vi "Set Command Factory.vi"(10 "commandFactory":refnum<class "Command Factory.lvclass">, 11 "Model in":refnum<class "Model.lvclass">) -> (3 "Model out":refnum<class "Model.lvclass">)   [LabVIEW 2015, in "Model.lvclass"]
uses:
  Model.lvclass
  Commands/Command Factory/Command Factory.lvclass
  Model.lvclass/Model.ctl
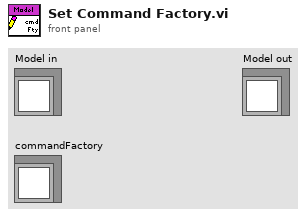
[diagram p1: front panel]
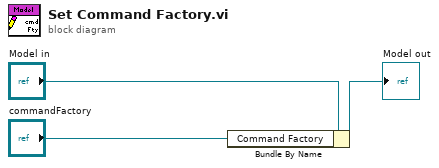
[diagram p0: block diagram]
diagram:
  n1 = Bundle By Name(cluster="Model in", "Command Factory"="commandFactory") -> (→"Model out":refnum<class "Model.lvclass">)
